vi "Process.vi"(8 "error in (no error)":errorcluster, 10 "Pound in":refnum<class "Pound.lvclass">, 11 "Qbus in":refnum<class "Qbus.lvclass">) -> (0 "error out":errorcluster)   [LabVIEW 2017, in "FileManager.lvlib"]
doc: "Manages TDMS data files from the time that the TDMS Creator process creates them until the Server Comm module successfully transfers them to NI InsightCM Server."
uses:
  <vilib>/addons/InsightCM/Devices/Shared/Common/FileManager/FileManager.lvlib
  <vilib>/addons/Qbus/Qbus.lvclass
  <vilib>/NI/Software Watchdog/Pound/Pound.lvclass
  <vilib>/addons/InsightCM/Devices/Shared/Common/FileManager/controls/config.ctl
  <vilib>/addons/TimerProcess/controls/taskType.ctl
  <vilib>/addons/TraceLogger/TraceLogger.lvlib
  <vilib>/NI/Software Watchdog/Watchdog/Watchdog.lvclass
  <vilib>/addons/TimerProcess/TimerProcess.lvlib
  <vilib>/addons/InsightCM/Devices/Shared/Common/ServerComm/ServerComm.lvlib
  <vilib>/addons/InsightCM/Utilities/GlobalConfiguration/GlobalConfiguration.lvlib
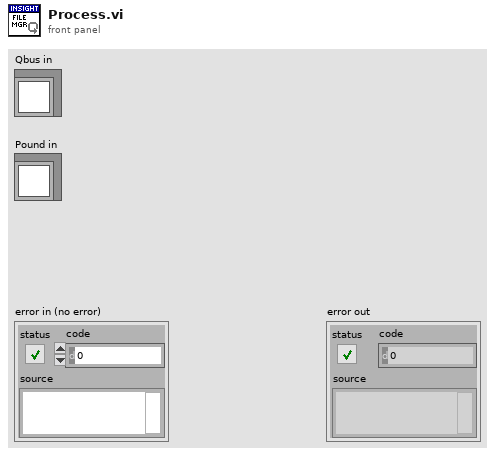
[diagram p1: front panel]
types:
  T1 = typedef "FileManager.lvlib/config.ctl" = cluster{"DataInProgress":variant, "InMemoryQ":refnum<queue>, "BacklogQ":refnum<queue>, "Online":bool, "Device":string, "Streams":variant, "MaxInMemFilesSize":i32, "MinDriveFreeSpace":i32, "Backlog TrendPts":bool, "Backlog Stream TrendPts":bool, "Backlog Extra Large Files":bool, "BacklogBatchSize":i32, "manage drive interval (sec)":dbl, "backlog file interval (sec)":dbl, "clean up folders interval (sec)":dbl}
  T2 = typedef "TimerProcess.lvlib/taskType.ctl" = enum16{"single", "repeat"}
  T3 = typedef "R2_Device.ctl" = cluster{"Id":string, "Name":string, "DeviceType":string, "HardwareName":string, "IpAddress":string, "HardwareInfo":T4[], "ApplicationType":string, "ApplicationVersion":string, "EquipmentIds":string[], "ConfigurationVersion":string, "State":T5, "Properties":T4[], "DataGroups":T6[], "BurstModeTrigger":T10, "SensorGroups":T11[], "Endpoints":T12[]}
  T4 = typedef "KeyValuePair.ctl" = cluster{"Key":string, "Value":string}
  T5 = typedef "DeviceState.ctl" = cluster{"Disabled":bool}
  T6 = typedef "R2_DataGroup.ctl" = cluster{"Name":string, "OperatingStates":T7[], "Properties":T4[], "EquipmentIds":string[], "AssetNodeId":string}
  T7 = typedef "OperatingState.ctl" = cluster{"Name":string, "Properties":T4[], "Triggers":T8[]}
  T8 = typedef "Trigger.ctl" = cluster{"Type":string, "Expression":string, "Conditions":T9[]}
  T9 = typedef "Condition.ctl" = cluster{"Source":string, "Type":string, "Operator":string, "CompareTo":string, "DwellSeconds":dbl}
  T10 = typedef "BurstModeTrigger.ctl" = cluster{"Trigger":T8, "SampleRate":string, "AcquisitionLength":string}
  T11 = typedef "DeviceSensorGroup.ctl" = cluster{"EquipId":string, "SensorGroupId":string}
  T12 = typedef "WirelessEndpoint.ctl" = cluster{"SerialNumber":string, "Properties":T4[], "Channels":T13[]}
  T13 = typedef "WirelessChannel.ctl" = cluster{"ChannelNumber":i32, "AssetId":string}
  T14 = typedef "SectionKeyValues.ctl" = cluster{"Section":string, "KeyValues":T4[]}
  T15 = typedef "FileManager.lvlib/SendEventRefRoutedMessage.ctl" = cluster{"event reference":T16, "DataGroup":string, "OperatingState":string, "StreamId":string, "LastBlock":bool, "TrendPoints Only":bool, "ExtraLargeFile":bool}
  T16 = typedef "DataEvent.lvlib/EventReference.ctl" = refnum<data-value>
  T17 = typedef "ServerComm.lvlib/ConnectionStatus.ctl" = enum16{"Offline", "NotAuthorized", "Online"}
  T18 = typedef "FileManager.lvlib/DataType.ctl" = enum16{"Default", "File", "InMemory", "EventRef", "EventRefFile"}
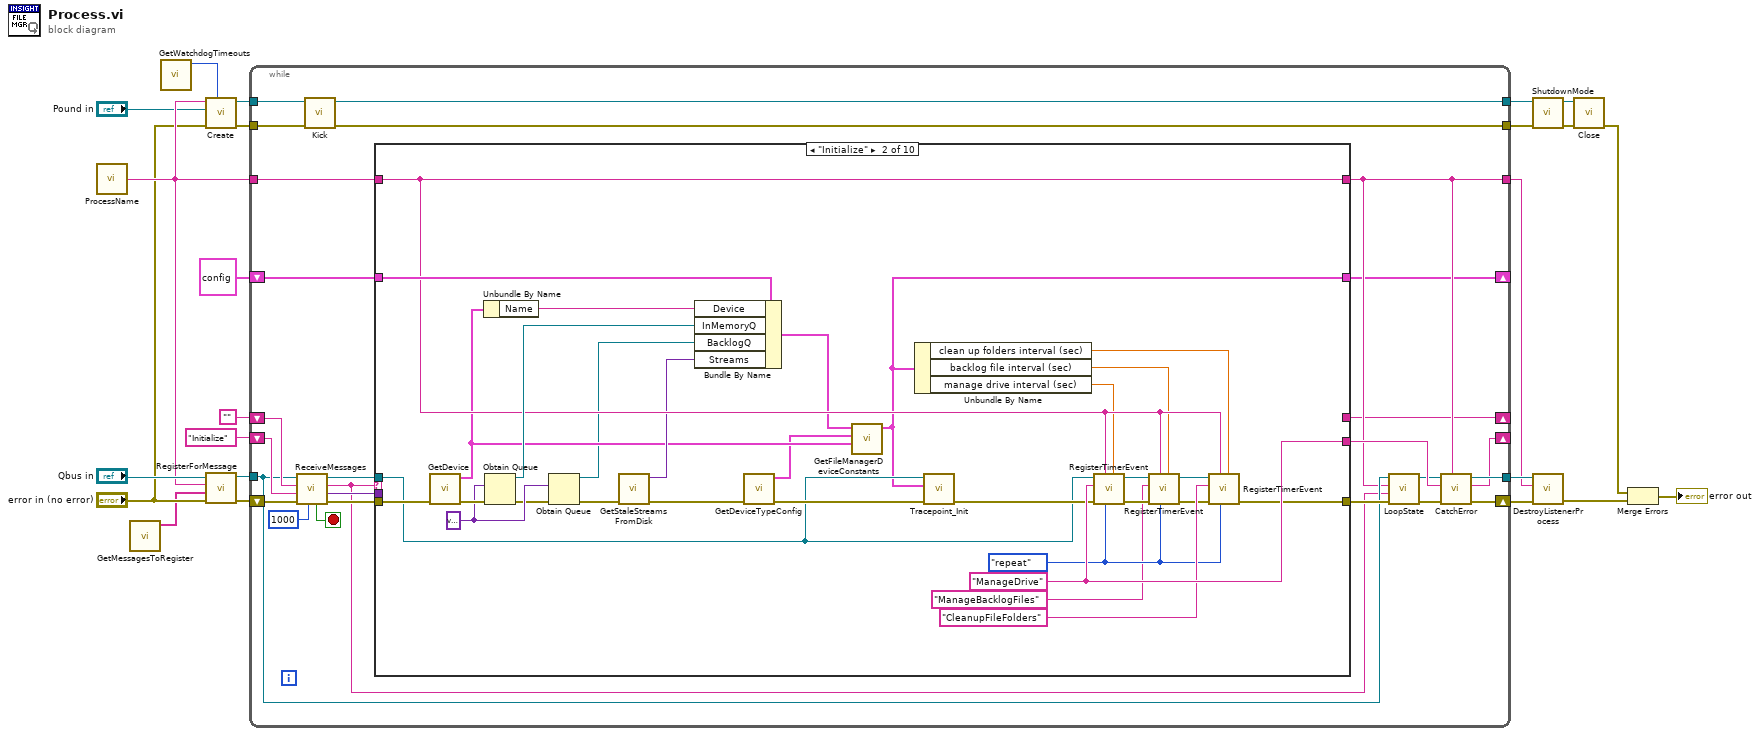
[diagram p0: block diagram]
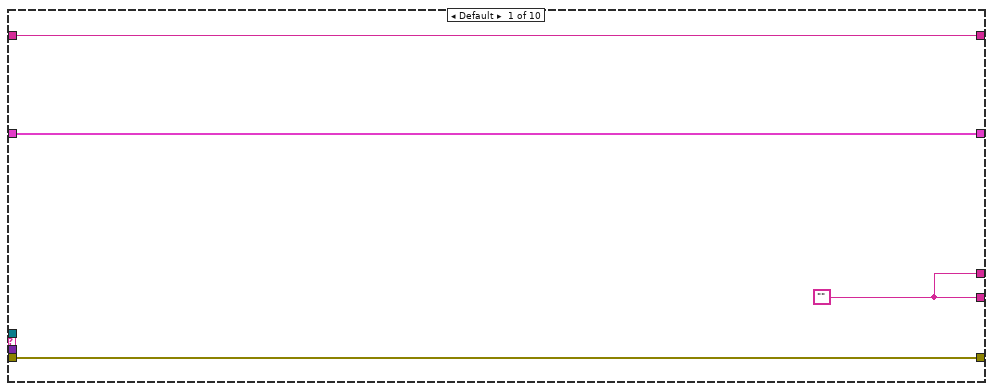
[diagram p2: hidden frame]
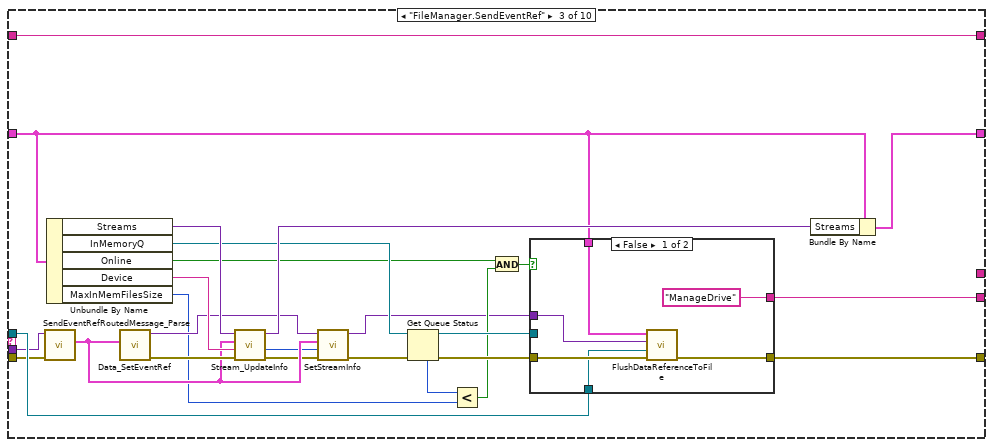
[diagram p3: hidden frame]
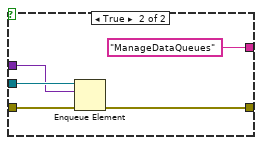
[diagram p4: hidden frame]
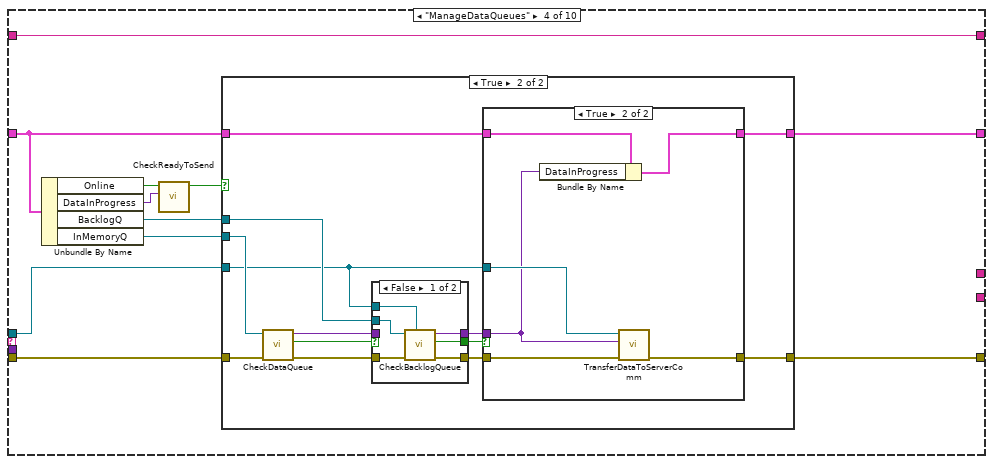
[diagram p5: hidden frame]
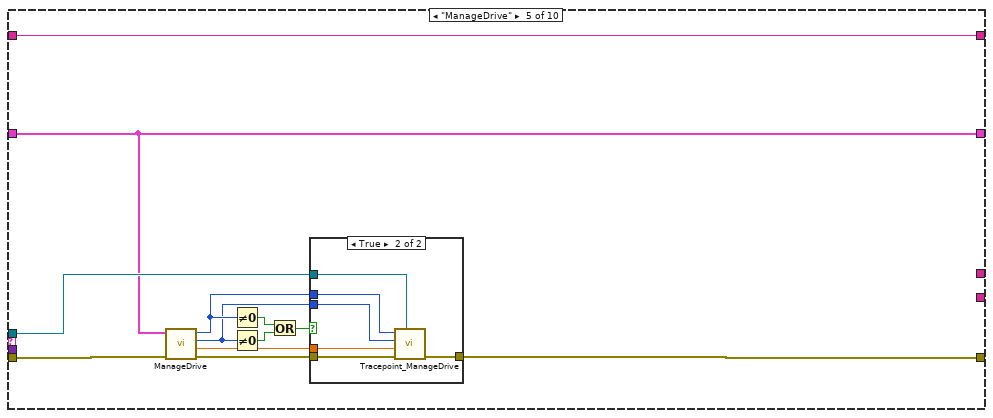
[diagram p9: hidden frame]
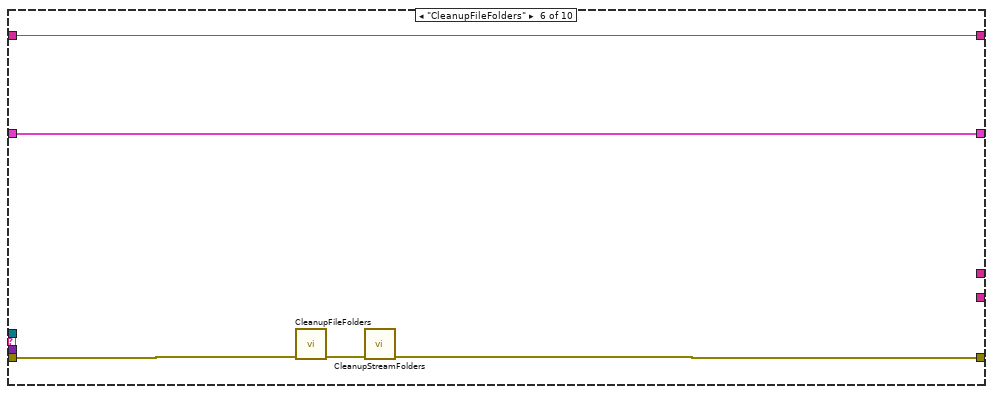
[diagram p11: hidden frame]
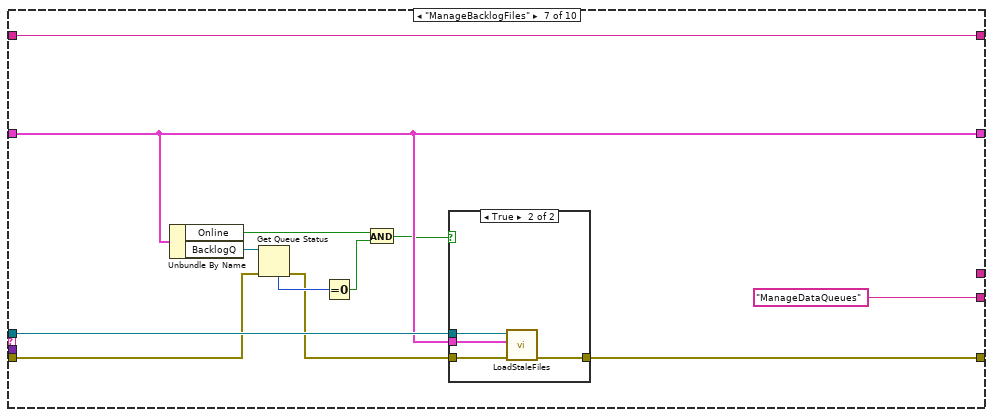
[diagram p12: hidden frame]
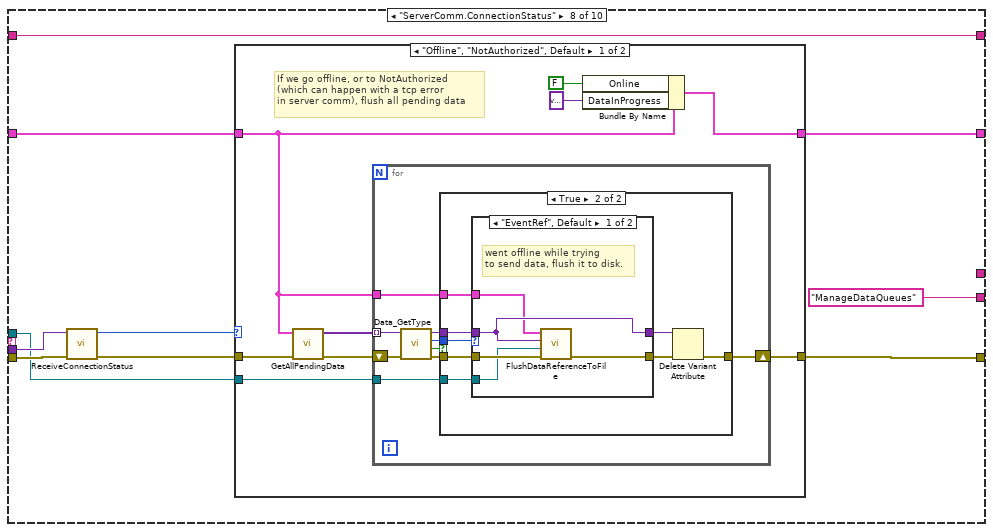
[diagram p14: hidden frame]
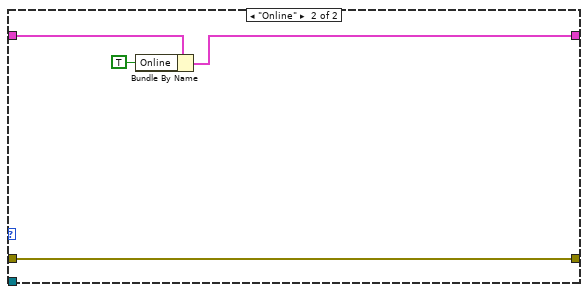
[diagram p17: hidden frame]
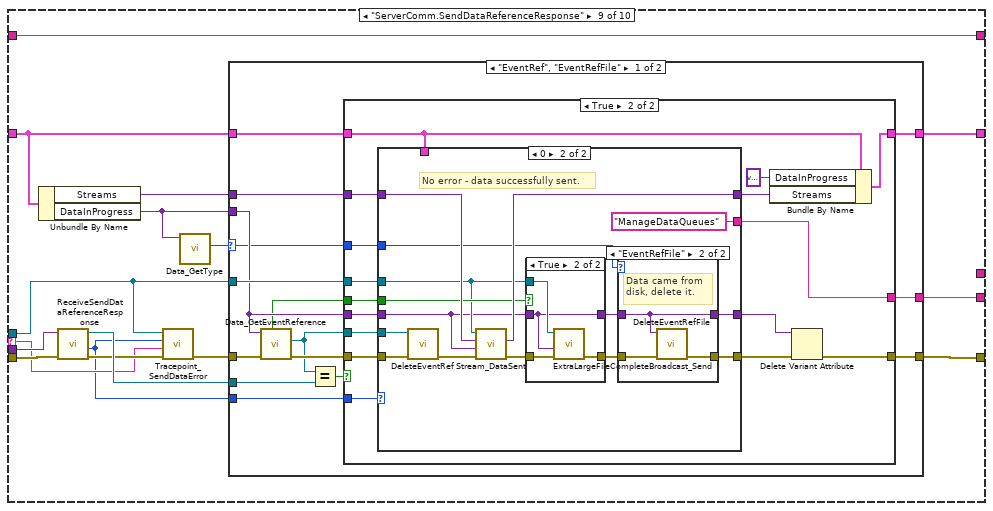
[diagram p18: hidden frame]
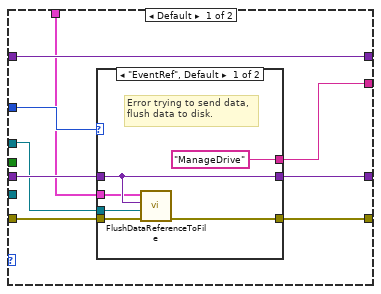
[diagram p20: hidden frame]
diagram:
  n1 = call <vilib>:"ProcessName.vi"() -> ("process name"=w14:string)  [unwired: 5 in]
  n2 = call <vilib>:"GetMessagesToRegister.vi"() -> ("subscribed messages"=w2:string[])  [unwired: 11 in]
  n3 = call <vilib>:"GetWatchdogTimeouts.vi"() -> ("software timeout"=w1:u32)  [unwired: 10 in, 1 out]
  n4 = call <vilib>:"Create.vi"("Execution Timeout (ms)"=w1, "error in (no error)"="error in (no error)", "Pound"="Pound in", "Name"=w14) -> ("error out"=w8:errorcluster, "Watchdog"=w13:refnum<data-value>)  [unwired: 6 in]
  n5 = call <vilib>:"RegisterForMessage.vi"("error in (no error)"="error in (no error)", "message names"=w2, "process name"=w14, "Qbus in"="Qbus in") -> ("error in (no error)"=w22:errorcluster, "Qbus out"=w21:refnum<class "Qbus.lvclass">)  [unwired: 6 in]
  n6 = while {
    shift-right: [w26] -> _
    shift-left: "" -> [w48]
    tunnel: w21 -> [w39]
    tunnel: w14 -> [w28]
    tunnel: [w42] -> w19
    tunnel: [w27] -> w18
    shift-right: [w41] -> _
    shift-left: "Initialize" -> [w44]
    shift-right: [w24] -> _
    shift-left: T1 {"DataInProgress"=variant, "InMemoryQ"=refnum, "BacklogQ"=refnum, "Online"=FALSE, "Device"="", "Streams"=variant, "MaxInMemFilesSize"=0, "MinDriveFreeSpace"=0, "Backlog TrendPts"=FALSE, "Backlog Stream TrendPts"=FALSE, "Backlog Extra Large Files"=FALSE, "BacklogBatchSize"=0, "manage drive interval (sec)"=0.0, "backlog file interval (sec)"=0.0, "clean up folders interval (sec)"=0.0} ("config") -> [w25]
    tunnel: w13 -> [w38]
    tunnel: [w37] -> w10
    tunnel: w8 -> [w36]
    tunnel: [w34] -> w7
    shift-right: [w43] -> w20
    shift-left: w22 -> [w35]
    stop <- w49 stop-if-true
    n7 = call <vilib>:"ReceiveMessages.vi"("timeout(1000)"=1000 ("Timeout(100)"), "error in (no error)"=w35, "priority action"=w44, "default action"=w48, "Qbus in"=w39) -> ("error out"=w47:errorcluster, "message value"=w45:variant, "action"=w32:string, "Qbus out"=w46:refnum<class "Qbus.lvclass">, "exit"=w49:bool)  [unwired: 2 in]
    n8 = call <vilib>:"Kick.vi"("error in (no error)"=w36, "Watchdog"=w38) -> ("error out"=w34:errorcluster, "Watchdog"=w37:refnum<data-value>)  [unwired: 8 in]
    n9 = case shown="\"Initialize\"" w32 {
      selector: w32 -> [_ _ _ _ _ _ _ _ w258 _]
      tunnel: w47 -> [w50 w81 w103 w128 w176 w187 w193 w214 w269 w349]
      tunnel: w46 -> [_ w65 w104 w126 w167 _ w197 w206 w259 _]
      tunnel: [w50 w68 w106 w124 w173 w185 w198 w210 w265 w349] -> w40
      tunnel: w45 -> [_ _ w102 _ _ _ _ w207 w268 _]
      tunnel: w25 -> [w51 w84 w85 w127 w165 w188 w196 w212 w256 w351]
      tunnel: [w51 w55 w110 w125 w165 w188 w196 w215 w264 w351] -> w24
      tunnel: [w52 w82 w86 _ _ _ "ManageDataQueues" ("MessageName") "ManageDataQueues" ("MessageName") w266 _] -> w33
      tunnel: w28 -> [w53 w75 w105 w123 w175 w186 w200 w211 w262 w350]
      tunnel: [w53 w75 w105 w123 w175 w186 w200 w211 w262 w350] -> w27
      tunnel: [w52 _ _ _ _ _ _ _ _ _] -> w26
      frame Default {
        w52 = ""
      }
      frame "Initialize" {
        w74 = taskType."repeat" ("type")
        w82 = "ManageDrive" ("callback action")
        w63 = variant
        n10 = call <vilib>:"GetDevice.vi"("error in (no error)"=w81) -> ("error out"=w70:errorcluster, "device configuration"=w64:T3)  [unwired: 8 in, 1 out]
        n11 = Unbundle By Name(w64) -> ("Name"=w72:string)
        n12 = Obtain Queue(element data type=w63, error in (no error)=w70) -> (queue out=w80:refnum<queue>, error out=w61:errorcluster)  [unwired: 3 in, 1 out]
        n13 = Obtain Queue(element data type=w63, error in (no error)=w61) -> (queue out=w60:refnum<queue>, error out=w62:errorcluster)  [unwired: 3 in, 1 out]
        n14 = call <vilib>:"GetStaleStreamsFromDisk.vi"("error in (no error)"=w62) -> ("error out"=w69:errorcluster, "streams"=w71:variant)  [unwired: 9 in]
        n15 = Bundle By Name(cluster=w84, "Device"=w72, "InMemoryQ"=w80, "BacklogQ"=w60, "Streams"=w71) -> (w58:T1)
        n16 = call <vilib>:"GetDeviceTypeConfig.vi"("error in (no error)"=w69) -> ("error out"=w67:errorcluster, "key values"=w59:T14[])  [unwired: 8 in, 1 out]
        n17 = call <vilib>:"GetFileManagerDeviceConstants.vi"("device"=w64, "key values"=w59, "config"=w58) -> ("config out"=w55:T1)  [unwired: 8 in]
        n18 = Unbundle By Name(w55) -> ("clean up folders interval (sec)"=w57:dbl, "backlog file interval (sec)"=w54:dbl, "manage drive interval (sec)"=w56:dbl)
        n19 = call <vilib>:"Tracepoint_Init.vi"("error in (no error)"=w67, "config"=w55, "Qbus"=w65) -> ("error out"=w66:errorcluster)  [unwired: 8 in]
        n20 = call <vilib>:"RegisterTimerEvent.vi"("interval (sec)"=w56, "type"=w74, "process name"=w75, "error in (no error)"=w66, "callback action"=w82, "qbus in"=w65) -> ("error out"=w77:errorcluster, "qbus out"=w83:refnum<class "Qbus.lvclass">)  [unwired: 4 in]
        n21 = call <vilib>:"RegisterTimerEvent.vi"("interval (sec)"=w54, "type"=w74, "process name"=w75, "error in (no error)"=w77, "callback action"="ManageBacklogFiles", "qbus in"=w83) -> ("error out"=w76:errorcluster, "qbus out"=w78:refnum<class "Qbus.lvclass">)  [unwired: 4 in]
        n22 = call <vilib>:"RegisterTimerEvent.vi"("interval (sec)"=w57, "type"=w74, "process name"=w75, "error in (no error)"=w76, "callback action"="CleanupFileFolders" ("TaskName"), "qbus in"=w78) -> ("error out"=w68:errorcluster)  [unwired: 4 in, 1 out]
      }
      frame "FileManager.SendEventRef" {
        n23 = call <vilib>:"SendEventRefRoutedMessage_Parse.vi"("error in (no error)"=w103, "message"=w102) -> ("SendEventRef"=w92:T15)  [unwired: 8 in, 1 out]
        n24 = Unbundle By Name(w85) -> ("Streams"=w101:variant, "InMemoryQ"=w98:refnum<queue>, "Online"=w95:bool, "Device"=w94:string, "MaxInMemFilesSize"=w87:i32)
        n25 = call <vilib>:"Data_SetEventRef.vi"("SendEventRef"=w92) -> ("error out"=w99:errorcluster, "data"=w93:variant)  [unwired: 7 in, 2 out]
        n26 = call <vilib>:"Stream_UpdateInfo.vi"("error in (no error)"=w99, "Device"=w94, "SendEventRef"=w92, "streams in"=w101) -> ("error out"=w90:errorcluster, "block number"=w91:i32, "streams out"=w100:variant)  [unwired: 5 in]
        n27 = call <vilib>:"SetStreamInfo.vi"("error in (no error)"=w90, "block"=w91, "SendEventRef"=w92, "data in"=w93) -> ("error out"=w89:errorcluster, "data out"=w88:variant)  [unwired: 6 in]
        n28 = Get Queue Status(queue=w98, error in (no error)=w89) -> (queue out=w107:refnum<queue>, error out=w108:errorcluster, # elements in queue=w109:i32)  [unwired: 1 in, 5 out]
        n29 = Less?(x=w109, y=w87) -> (x < y?=w96:bool)
        n30 = And(x=w95, y=w96) -> (x .and. y?=w97:bool)
        n31 = case shown="False" w97 {
          tunnel: [w115 w121] -> w106
          tunnel: w108 -> [w116 w120]
          tunnel: w107 -> [_ w119]
          tunnel: w88 -> [w114 w118]
          tunnel: w104 -> [w113 _]
          tunnel: ["ManageDrive" ("MessageName") "ManageDataQueues" ("MessageName")] -> w86
          tunnel: w85 -> [w111 _]
          frame False {
            n32 = call <vilib>:"FlushDataReferenceToFile.vi"("error in (no error)"=w116, "Qbus"=w113, "data"=w114, "config"=w111) -> ("error out"=w115:errorcluster)  [unwired: 7 in]
          }
          frame True {
            n33 = Enqueue Element(queue=w119, element=w118, error in (no error)=w120) -> (error out=w121:errorcluster)  [unwired: 1 in, 2 out]
          }
        }
        n34 = Bundle By Name(cluster=w85, "Streams"=w100) -> (w110:T1)
      }
      frame "ManageDataQueues" {
        n35 = Unbundle By Name(w127) -> ("Online"=w132:bool, "DataInProgress"=w131:variant, "BacklogQ"=w122:refnum<queue>, "InMemoryQ"=w129:refnum<queue>)
        n36 = call <vilib>:"CheckReadyToSend.vi"("data in progress"=w131, "online"=w132) -> ("read to send"=w130:bool)  [unwired: 9 in]
        n37 = case shown="True" w130 {
          tunnel: w129 -> [_ w143]
          tunnel: w128 -> [w134 w144]
          tunnel: w127 -> [w133 w147]
          tunnel: w126 -> [_ w138]
          tunnel: [w133 w146] -> w125
          tunnel: [w134 w145] -> w124
          tunnel: w122 -> [_ w139]
          frame False {
          }
          frame True {
            n38 = call <vilib>:"CheckDataQueue.vi"("error in (no error)"=w144, "data Q"=w143) -> ("error out"=w137:errorcluster, "ready"=w136:bool, "data"=w135:variant)  [unwired: 7 in]
            n39 = case shown="False" w136 {
              selector: w136 -> [_ w156]
              tunnel: [w150 w156] -> w142
              tunnel: [w151 w155] -> w141
              tunnel: w135 -> [_ w155]
              tunnel: [w149 w154] -> w140
              tunnel: w137 -> [w152 w154]
              tunnel: w139 -> [w153 _]
              tunnel: w138 -> [w148 _]
              frame False {
                n40 = call <vilib>:"CheckBacklogQueue.vi"("Qbus"=w148, "error in (no error)"=w152, "BacklogQ"=w153) -> ("error out"=w149:errorcluster, "ready"=w150:bool, "data"=w151:variant)  [unwired: 6 in]
              }
              frame True {
              }
            }
            n41 = case shown="True" w142 {
              tunnel: w147 -> [w158 w164]
              tunnel: w140 -> [w157 w163]
              tunnel: w138 -> [_ w160]
              tunnel: [w158 w162] -> w146
              tunnel: [w157 w161] -> w145
              tunnel: w141 -> [_ w159]
              frame False {
              }
              frame True {
                n42 = Bundle By Name(cluster=w164, "DataInProgress"=w159) -> (w162:T1)
                n43 = call <vilib>:"TransferDataToServerComm.vi"("error in (no error)"=w163, "data"=w159, "Qbus"=w160) -> ("error out"=w161:errorcluster)  [unwired: 8 in]
              }
            }
          }
        }
      }
      frame "ManageDrive" {
        n44 = call <vilib>:"ManageDrive.vi"("error in (no error)"=w176, "config"=w165) -> ("error out"=w174:errorcluster, "free disk space"=w166:dbl, "streams deleted"=w168:i32, "files deleted"=w169:i32)  [unwired: 6 in]
        n45 = Not Equal To 0?(x=w169) -> (x != 0?=w172:bool)
        n46 = Not Equal To 0?(x=w168) -> (x != 0?=w171:bool)
        n47 = Or(x=w172, y=w171) -> (x .or. y?=w170:bool)
        n48 = case shown="True" w170 {
          tunnel: w174 -> [w177 w183]
          tunnel: [w177 w182] -> w173
          tunnel: w169 -> [_ w180]
          tunnel: w168 -> [_ w179]
          tunnel: w167 -> [_ w181]
          tunnel: w166 -> [_ w178]
          frame False {
          }
          frame True {
            n49 = call <vilib>:"Tracepoint_ManageDrive.vi"("Qbus in"=w181, "error in (no error)"=w183, "free disk space"=w178, "streams deleted"=w179, "files deleted"=w180) -> ("error out"=w182:errorcluster)  [unwired: 6 in]
          }
        }
      }
      frame "CleanupFileFolders" {
        n50 = call <vilib>:"CleanupFileFolders.vi"("error in (no error)"=w187) -> ("error out"=w184:errorcluster)  [unwired: 10 in]
        n51 = call <vilib>:"CleanupStreamFolders.vi"("error in (no error)"=w184) -> ("error out"=w185:errorcluster)  [unwired: 10 in]
      }
      frame "ManageBacklogFiles" {
        n52 = Unbundle By Name(w196) -> ("Online"=w191:bool, "BacklogQ"=w195:refnum<queue>)
        n53 = Get Queue Status(queue=w195, error in (no error)=w193) -> (error out=w192:errorcluster, # elements in queue=w194:i32)  [unwired: 1 in, 6 out]
        n54 = Equal To 0?(x=w194) -> (x = 0?=w190:bool)
        n55 = And(x=w191, y=w190) -> (x .and. y?=w189:bool)
        n56 = case shown="True" w189 {
          tunnel: w192 -> [w201 w205]
          tunnel: [w201 w204] -> w198
          tunnel: w197 -> [_ w203]
          tunnel: w196 -> [_ w202]
          frame False {
          }
          frame True {
            n57 = call <vilib>:"LoadStaleFiles.vi"("error in (no error)"=w205, "config"=w202, "Qbus"=w203) -> ("error out"=w204:errorcluster)  [unwired: 8 in]
          }
        }
      }
      frame "ServerComm.ConnectionStatus" {
        n58 = call <vilib>:"ReceiveConnectionStatus.vi"("error in (no error)"=w214, "body"=w207) -> ("error out"=w209:errorcluster, "status"=w208:T17)  [unwired: 6 in, 2 out]
        n59 = case shown="\"Offline\", \"NotAuthorized\", Default" w208 {
          tunnel: [w223 w253] -> w215
          tunnel: w212 -> [w216 w252]
          tunnel: [w221 w251] -> w210
          tunnel: w209 -> [w217 w251]
          tunnel: w206 -> [w220 _]
          frame "Offline", "NotAuthorized", Default {
            # "If we go offline, or to NotAuthorized\n(which can happen with a tcp error\nin server comm), flush all pending data"
            n60 = call <vilib>:"GetAllPendingData.vi"("error in (no error)"=w217, "config"=w216) -> ("error out"=w218:errorcluster, "all pending data"=w219:variant[])  [unwired: 8 in]
            n61 = for {
              tunnel: w220 -> [w230]
              shift-right: [w231] -> w221
              shift-left: w218 -> [w233]
              tunnel: w219 -> [w226] mode=indexing
              tunnel: w216 -> [w225]
              n62 = call <vilib>:"Data_GetType.vi"("error in"=w233, "data"=w226) -> ("error out"=w232:errorcluster, "in progress"=w227:bool, "type"=w228:T18, "data out"=w229:variant)  [unwired: 6 in]
              n63 = case shown="True" w227 {
                tunnel: w232 -> [w234 w242]
                tunnel: [w234 w237] -> w231
                tunnel: w230 -> [_ w241]
                tunnel: w229 -> [_ w240]
                tunnel: w228 -> [_ w239]
                tunnel: w225 -> [_ w235]
                frame False {
                }
                frame True {
                  n64 = case shown="\"EventRef\", Default" w239 {
                    tunnel: w242 -> [w247 w249]
                    tunnel: w240 -> [w244 w248]
                    tunnel: [w246 w249] -> w238
                    tunnel: w241 -> [w245 _]
                    tunnel: [w244 w248] -> w236
                    tunnel: w235 -> [w243 _]
                    frame "EventRef", Default {
                      # "went offline while trying \nto send data, flush it to disk."
                      n65 = call <vilib>:"FlushDataReferenceToFile.vi"("error in (no error)"=w247, "Qbus"=w245, "data"=w244, "config"=w243) -> ("error out"=w246:errorcluster)  [unwired: 7 in]
                    }
                    frame "EventRefFile" {
                      # "went offline while  trying to\nsend data, it was loaded \nfrom disk and is still there."
                    }
                  }
                  n66 = Delete Variant Attribute(4:w238, 7:w236) -> (0:w237:errorcluster)  [unwired: 1 in, 2 out]
                }
              }
            }
            n67 = Bundle By Name(cluster=w216, "Online"=FALSE, "DataInProgress"=variant) -> (w223:T1)
          }
          frame "Online" {
            n68 = Bundle By Name(cluster=w252, "Online"=TRUE) -> (w253:T1)
          }
        }
      }
      frame "ServerComm.SendDataReferenceResponse" {
        n69 = Unbundle By Name(w256) -> ("Streams"=w263:variant, "DataInProgress"=w255:variant)
        n70 = call <vilib>:"ReceiveSendDataReferenceResponse.vi"("error in (no error)"=w269, "body"=w268) -> ("error out"=w261:errorcluster, "error code"=w257:i32, "event reference"=w267:T16)  [unwired: 6 in, 1 out]
        n71 = call <vilib>:"Tracepoint_SendDataError.vi"("error in (no error)"=w261, "message"=w258, "error code"=w257, "Qbus"=w259) -> ("error out"=w260:errorcluster)  [unwired: 7 in]
        n72 = call <vilib>:"Data_GetType.vi"("data"=w255) -> ("type"=w254:T18)  [unwired: 7 in, 3 out]
        n73 = case shown="\"EventRef\", \"EventRefFile\"" w254 {
          selector: w254 -> [w272 _]
          tunnel: w260 -> [w275 w347]
          tunnel: w255 -> [w274 _]
          tunnel: w267 -> [w284 _]
          tunnel: w257 -> [w282 _]
          tunnel: w256 -> [w281 w348]
          tunnel: [w280 _] -> w266
          tunnel: [w279 w347] -> w265
          tunnel: [w278 w348] -> w264
          tunnel: w259 -> [w277 _]
          tunnel: w263 -> [w276 _]
          frame "EventRef", "EventRefFile" {
            n74 = call <vilib>:"Data_GetEventReference.vi"("error in (no error)"=w275, "data"=w274) -> ("error out"=w273:errorcluster, "event reference"=w271:T16, "extra large file"=w270:bool)  [unwired: 4 in, 3 out]
            n75 = Equal?(x=w271, y=w284) -> (x = y?=w283:bool)
            n76 = case shown="True" w283 {
              tunnel: w282 -> [_ w295]
              tunnel: w273 -> [w285 w302]
              tunnel: w271 -> [_ w301]
              tunnel: w281 -> [w286 w288]
              tunnel: w274 -> [_ w299]
              tunnel: [_ w289] -> w280
              tunnel: [w285 w291] -> w279
              tunnel: [w286 w298] -> w278
              tunnel: w277 -> [_ w297]
              tunnel: w276 -> [_ w294]
              tunnel: w272 -> [_ w293]
              tunnel: w270 -> [_ w287]
              frame False {
              }
              frame True {
                n77 = case shown="0" w295 {
                  tunnel: w302 -> [w311 w335]
                  tunnel: w301 -> [_ w334]
                  tunnel: w299 -> [w310 w321]
                  tunnel: [w307 w329] -> w292
                  tunnel: w297 -> [w308 w323]
                  tunnel: w294 -> [w309 w331]
                  tunnel: [w309 w332] -> w296
                  tunnel: w293 -> [w306 w330]
                  tunnel: [w305 w328] -> w290
                  tunnel: [w304 "ManageDataQueues" ("MessageName")] -> w289
                  tunnel: w288 -> [w303 _]
                  tunnel: w287 -> [_ w324]
                  frame Default {
                    n78 = case shown="\"EventRef\", Default" w306 {
                      tunnel: w311 -> [w317 w320]
                      tunnel: w310 -> [w314 w319]
                      tunnel: w308 -> [w316 _]
                      tunnel: [w315 w320] -> w307
                      tunnel: [w314 w319] -> w305
                      tunnel: ["ManageDrive" ("MessageName") "ManageDataQueues" ("MessageName")] -> w304
                      tunnel: w303 -> [w312 _]
                      frame "EventRef", Default {
                        # "Error trying to send data,\nflush data to disk."
                        n79 = call <vilib>:"FlushDataReferenceToFile.vi"("error in (no error)"=w317, "Qbus"=w316, "data"=w314, "config"=w312) -> ("error out"=w315:errorcluster)  [unwired: 7 in]
                      }
                      frame "EventRefFile" {
                        # "Error trying to send data,\nit was loaded from disk and\nis still there."
                      }
                    }
                  }
                  frame 0 {
                    # "No error - data successfully sent."
                    n80 = call <vilib>:"DeleteEventRef.vi"("error in (no error)"=w335, "event ref"=w334) -> ("error out"=w333:errorcluster)  [unwired: 9 in]
                    n81 = call <vilib>:"Stream_DataSent.vi"("error in (no error)"=w333, "data"=w321, "streams"=w331, "Qbus"=w323) -> ("error out"=w326:errorcluster, "streams out"=w332:variant)  [unwired: 6 in]
                    n82 = case shown="True" w324 {
                      tunnel: w326 -> [w337 w341]
                      tunnel: [w337 w340] -> w325
                      tunnel: w323 -> [_ w339]
                      tunnel: [w336 w338] -> w322
                      tunnel: w321 -> [w336 w338]
                      frame False {
                      }
                      frame True {
                        n83 = call <vilib>:"ExtraLargeFileCompleteBroadcast_Send.vi"("error in (no error)"=w341, "data"=w338, "Qbus in"=w339) -> ("error out"=w340:errorcluster)  [unwired: 8 in]
                      }
                    }
                    n84 = case shown="\"EventRefFile\"" w330 {
                      tunnel: w325 -> [w343 w346]
                      tunnel: [w343 w345] -> w329
                      tunnel: w322 -> [w342 w344]
                      tunnel: [w342 w344] -> w328
                      frame Default {
                      }
                      frame "EventRefFile" {
                        # "Data came from\ndisk, delete it."
                        n85 = call <vilib>:"DeleteEventRefFile.vi"("error in (no error)"=w346, "data"=w344) -> ("error out"=w345:errorcluster)  [unwired: 9 in]
                      }
                    }
                  }
                }
                n86 = Bundle By Name(cluster=w288, "DataInProgress"=variant, "Streams"=w296) -> (w298:T1)
                n87 = Delete Variant Attribute(4:w292, 7:w290) -> (0:w291:errorcluster)  [unwired: 1 in, 2 out]
              }
            }
          }
          frame Default {
          }
        }
      }
      frame "Exit" {
      }
    }
    n88 = call <vilib>:"LoopState.vi"("error in (no error)"=w40, "loop action"=w32, "process name"=w27, "Qbus in"=w39) -> ("error out"=w30:errorcluster, "Qbus out"=w29:refnum<class "Qbus.lvclass">)  [unwired: 6 in]
    n89 = call <vilib>:"CatchError.vi"("source"=w27, "error in (no error)"=w30, "next action in"=w33, "Qbus in"=w29) -> ("error out"=w43:errorcluster, "next action out"=w41:string, "Qbus out"=w42:refnum<class "Qbus.lvclass">)  [unwired: 5 in]
  }
  n90 = call <vilib>:"ShutdownMode.vi"("error in (no error)"=w7, "Watchdog"=w10) -> ("error out"=w9:errorcluster, "Watchdog"=w11:refnum<data-value>)  [unwired: 8 in]
  n91 = call <vilib>:"DestroyListenerProcess.vi"("error in (no error)"=w20, "process name"=w18, "Qbus in"=w19) -> ("error in (no error)"=w6:errorcluster)  [unwired: 7 in, 1 out]
  n92 = call <vilib>:"Close.vi"("error in (no error)"=w9, "Watchdog"=w11) -> ("error out"=w5:errorcluster)  [unwired: 9 in]
  n93 = Merge Errors(w5, w6) -> (→"error out":errorcluster)
